vi "BL132 CAM45.vi"() -> ()   [LabVIEW 2015]
panel:
  in  "error in":errorcluster
  out "error out":errorcluster
  out "x = y?":bool
  out "APX PREP TOP":T1(plugin-control)
  out "APX Sample Top View in PREP":T1(plugin-control)
  out "APX PREP SIDE":T1(plugin-control)
  out "APX Sample Side View in PREP":T1(plugin-control)
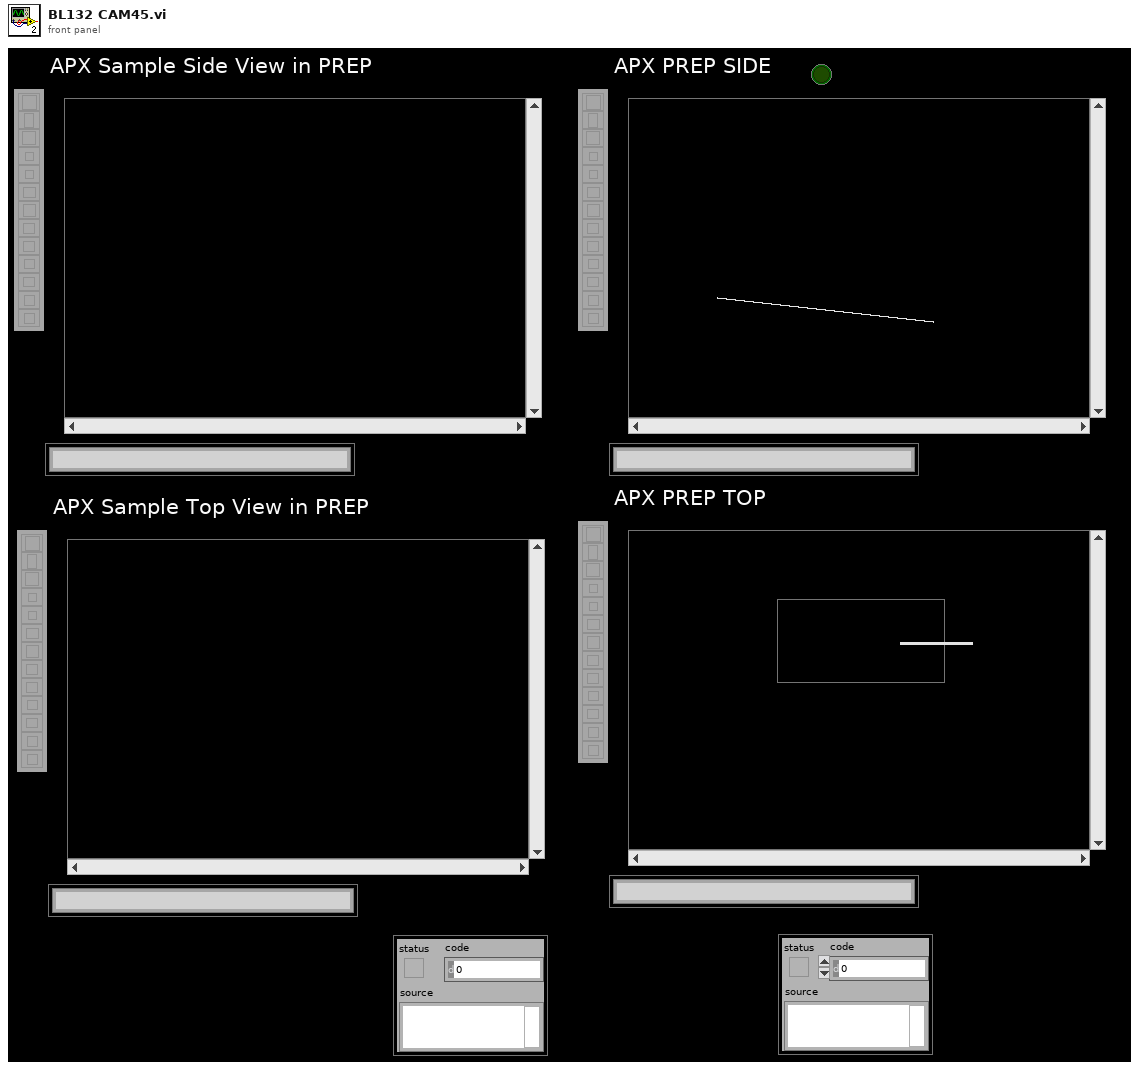
[diagram p1: front panel]
types:
  T1 = typedef "IMAQ Image.ctl" = refnum<image>
  T2 = cluster{"Pattern":i32, "Algorithm":i32, "Red Gain":dbl, "Green Gain":dbl, "Blue Gain":dbl}
  T3 = typedef "Image Type" = u32
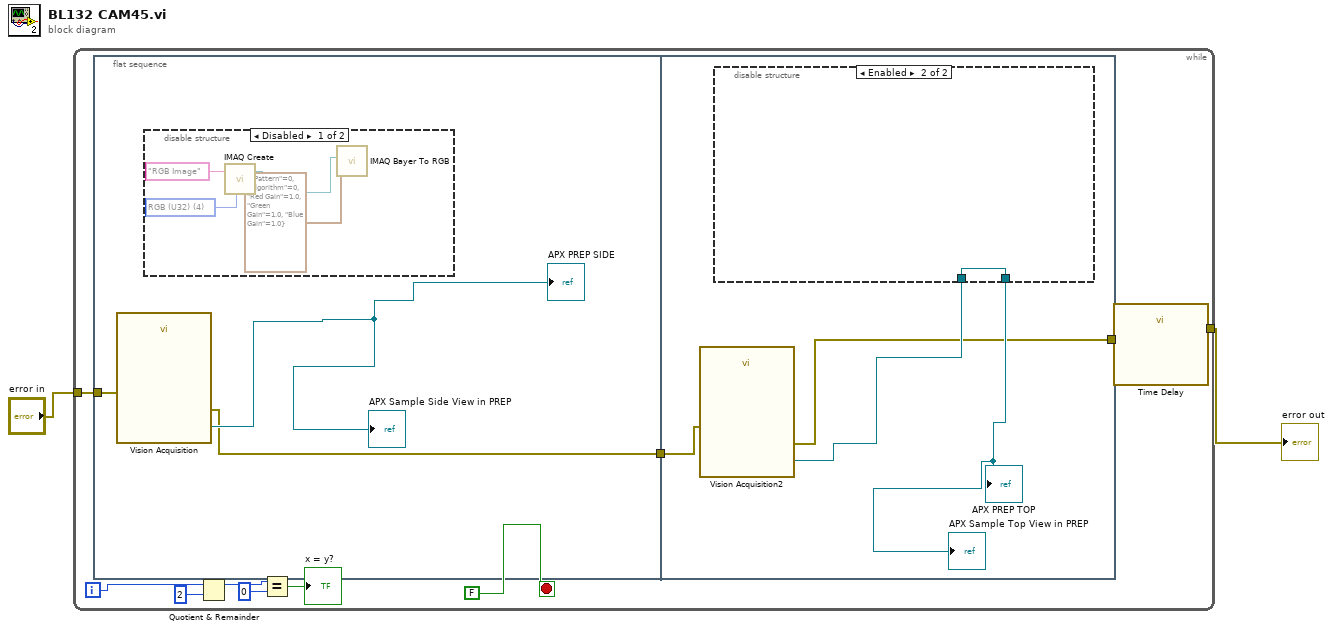
[diagram p0: block diagram]
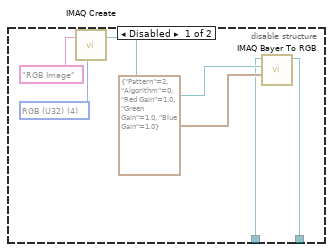
[diagram p3: hidden frame]
diagram:
  n1 = while {
    tunnel: "error in" -> [w5]
    tunnel: [w3] -> w1
    i -> [w11]
    stop <- FALSE stop-if-true
    n2 = flat-sequence {
      tunnel: [w14] -> w6
      tunnel: w5 -> [w13]
      tunnel: w6 -> [w21]
      tunnel: [w20] -> w4
      frame #0 {
        n3 = call "Vision Acquisition"("error in"=w13) -> ("Image Out"=→"APX Sample Side View in PREP" →"APX PREP SIDE":T1, "error out"=w14:errorcluster)  [unwired: 25 in]
        n4 = disable-structure shown="Disabled" {
          frame Disabled {
            w17 = T3 4 items=["Grayscale (U8)", "Grayscale (I16)", "Grayscale (SGL)", "Complex (CSG)", "RGB (U32)", "HSL (U32)", "RGB (U64)", "Grayscale (U16)"] ("Image Type")
            n5 = call "IMAQ Create"("Image Name"="RGB Image", "Image Type"=w17) -> ("New Image"=w16:T1)  [unwired: 2 in, 2 out]
            n6 = call "IMAQ Bayer To RGB"("Bayer Parameters"=T2 {"Pattern"=0, "Algorithm"=0, "Red Gain"=1.0, "Green Gain"=1.0, "Blue Gain"=1.0}, "Image Dst"=w16) -> ()  [unwired: 8 in, 2 out]
          }
          frame Enabled {
          }
        }
      }
      frame #1 {
        n7 = call "Vision Acquisition2"("error in"=w21) -> ("Image Out"=w23:T1, "error out"=w20:errorcluster)  [unwired: 25 in]
        n8 = disable-structure shown="Enabled" {
          disable-tunnel: w23 -> [w25 w30]
          disable-tunnel: [w24 w30] -> w22
          frame Disabled {
            w27 = T3 4 items=["Grayscale (U8)", "Grayscale (I16)", "Grayscale (SGL)", "Complex (CSG)", "RGB (U32)", "HSL (U32)", "RGB (U64)", "Grayscale (U16)"] ("Image Type")
            n9 = call "IMAQ Create"("Image Name"="RGB Image", "Image Type"=w27) -> ("New Image"=w26:T1)  [unwired: 2 in, 2 out]
            n10 = call "IMAQ Bayer To RGB"("Bayer Parameters"=T2 {"Pattern"=2, "Algorithm"=0, "Red Gain"=1.0, "Green Gain"=1.0, "Blue Gain"=1.0}, "Image Dst"=w26, "Image Src"=w25) -> ("Image Dst Out"=w24:T1)  [unwired: 7 in, 1 out]
          }
          frame Enabled {
          }
        }
        "APX Sample Top View in PREP" <- w22
        "APX PREP TOP" <- w22
      }
    }
    n11 = Quotient & Remainder(x=w11, y=2) -> (x-y*floor(x/y)=w9:i32)  [unwired: 1 out]
    n12 = Equal?(x=w9, y=0) -> (x = y?=→"x = y?":bool)
    n13 = call "Time Delay"("error in (no error)"=w4) -> ("error out"=w3:errorcluster)  [unwired: 10 in]
  }
  "error out" <- w1
